vi "to string.vi"(8 "error in":errorcluster, 11 "sample module configuration in":refnum<class "sample module configuration.lvclass">) -> (0 "error out":errorcluster, 1 "data":string, 2 "version":string, 3 "sample module configuration out":refnum<class "sample module configuration.lvclass">)   [LabVIEW 2013, in "sample module configuration.lvclass"]
doc: "Provides an interface for saving a module configuration to a file or other serialized data source. It is recommended that all children of this class store data in two sets--data required for its own initialization, and any data required for parent initialization--and that each implementation uses the <b>Call Parent Method</b> primitive to serialize parent information."
uses:
  sample module configuration.lvclass
  module configuration/TBM module configuration.lvclass
  sample module configuration.lvclass/sample module configuration.ctl
  channel/TBM channel.lvclass
  root configuration/TBM configuration.lvclass
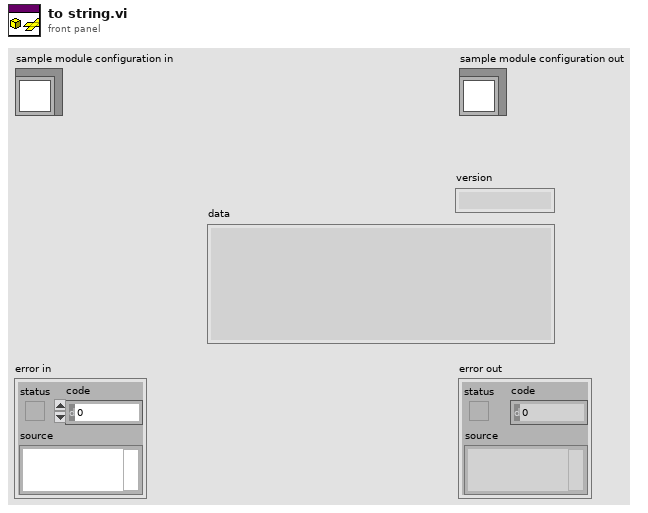
[diagram p1: front panel]
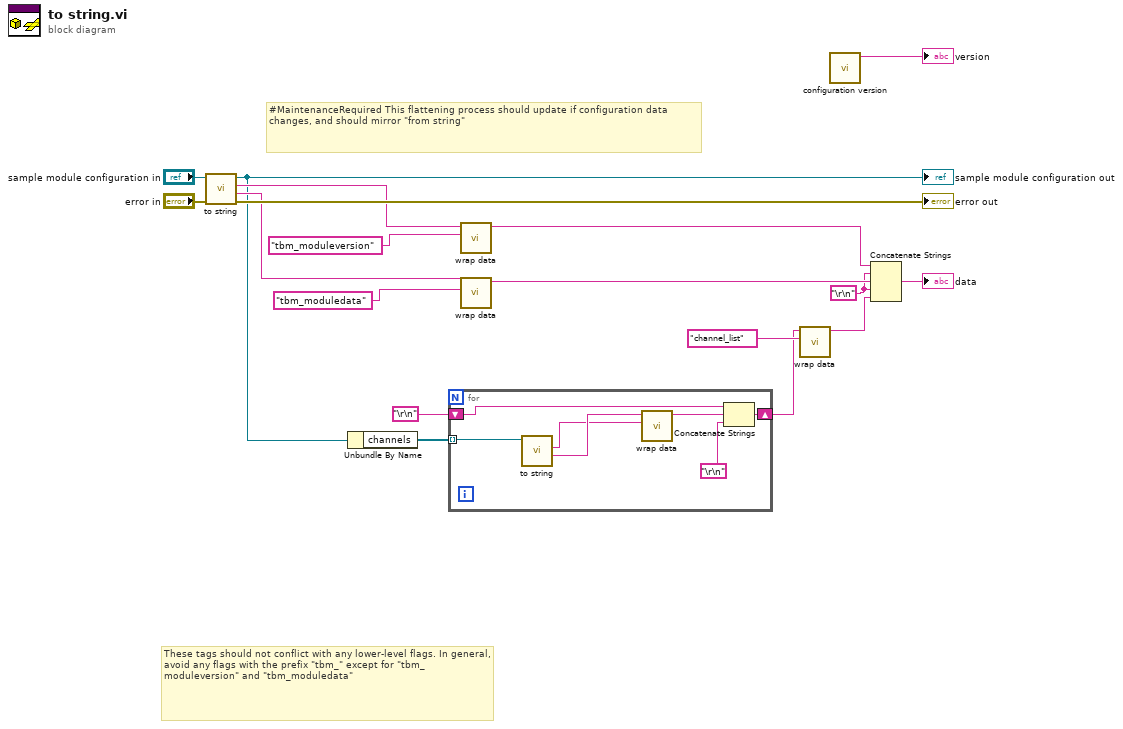
[diagram p0: block diagram]
diagram:
  w6 = "\r\n"
  # "These tags should not conflict with any lower-level flags. In general, avoid any flags with the prefix \"tbm_\" except for \"tbm_moduleversion\" and \"tbm_moduledata\""
  # "#MaintenanceRequired This flattening process should update if configuration data changes, and should mirror \"from string\""
  n1 = call-parent "to string.vi"("error in"="error in", "module configuration in"="sample module configuration in") -> ("error out"=→"error out":errorcluster, "data"=w12:string, "version"=w13:string, "module configuration out"=w11:refnum<class "sample module configuration.lvclass">)  [unwired: 6 in]
  "sample module configuration out" <- w11
  n2 = Unbundle By Name(w11) -> ("channels"=w5:refnum<class "TBM channel.lvclass">[])
  n3 = for {
    tunnel: w5 -> [w21] mode=indexing
    shift-right: [w25] -> w3
    shift-left: "\r\n" -> [w23]
    n4 = call-dynamic "to string.vi"("channel in"=w21) -> ("channel data"=w20:string, "identifier"=w19:string)  [unwired: 7 in, 2 out]
    n5 = call "wrap data.vi"("identifier"=w19, "data to wrap"=w20) -> ("wrapped data"=w22:string)  [unwired: 9 in]
    n6 = Concatenate Strings(w23, w22, "\r\n") -> (w25:string)
  }
  n7 = call "wrap data.vi"("identifier"="tbm_moduleversion" ("additional identifier"), "data to wrap"=w13) -> ("wrapped data"=w9:string)  [unwired: 9 in]
  n8 = call "wrap data.vi"("identifier"="tbm_moduledata" ("additional identifier"), "data to wrap"=w12) -> ("wrapped data"=w8:string)  [unwired: 9 in]
  n9 = call "wrap data.vi"("identifier"="channel_list" ("additional identifier"), "data to wrap"=w3) -> ("wrapped data"=w4:string)  [unwired: 9 in]
  n10 = call "configuration version.vi"() -> ("current version"=→"version":string)  [unwired: 11 in]
  n11 = Concatenate Strings(w9, w6, w8, w6, w4) -> (→"data":string)
